vi "Move to New Position.vi"(7 "Curr Filter":i32, 8 "error in (no error)":errorcluster, 9 "Target Filter":i32, 10 "Filter Wheel (0:n-1)":i32, 11 "FW Arduino Control in":refnum<class "FW Arduino Control.lvclass">) -> (0 "error out":errorcluster, 1 "Actual Distance":i32[](array[numeric]), 2 "Log":string, 3 "FW Arduino Control out":refnum<class "FW Arduino Control.lvclass">)   [LabVIEW 2024, in "FW Arduino Control.lvclass"]
uses:
  FW Arduino Control.lvclass
  C:/Development/Prime-RIMAS/Filter Wheel/Filter Wheel Object/Filter Wheel.lvclass
  FW Arduino Control.lvclass/FW Arduino Control.ctl
panel:
  out "notches":i32
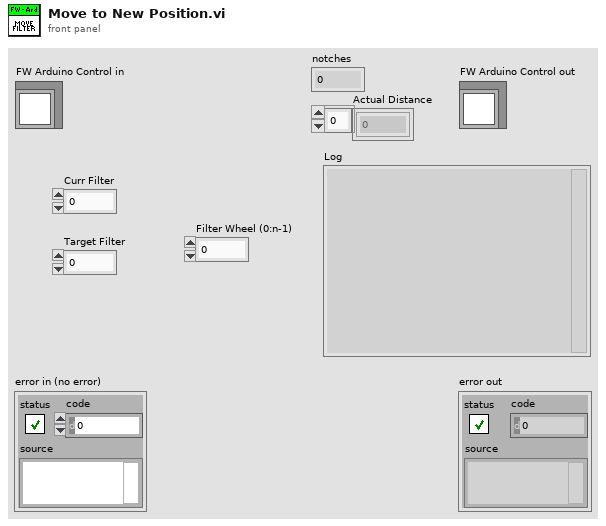
[diagram p1: front panel]
types:
  T1 = typedef "Filter Wheel Arduino Homing cluster.ctl" = cluster{"Direction (F: CW)":bool, "Speed":i32, "Accel":i32, "Min Distance":i32, "Short Leg":i32, "Error Cnts":i32}
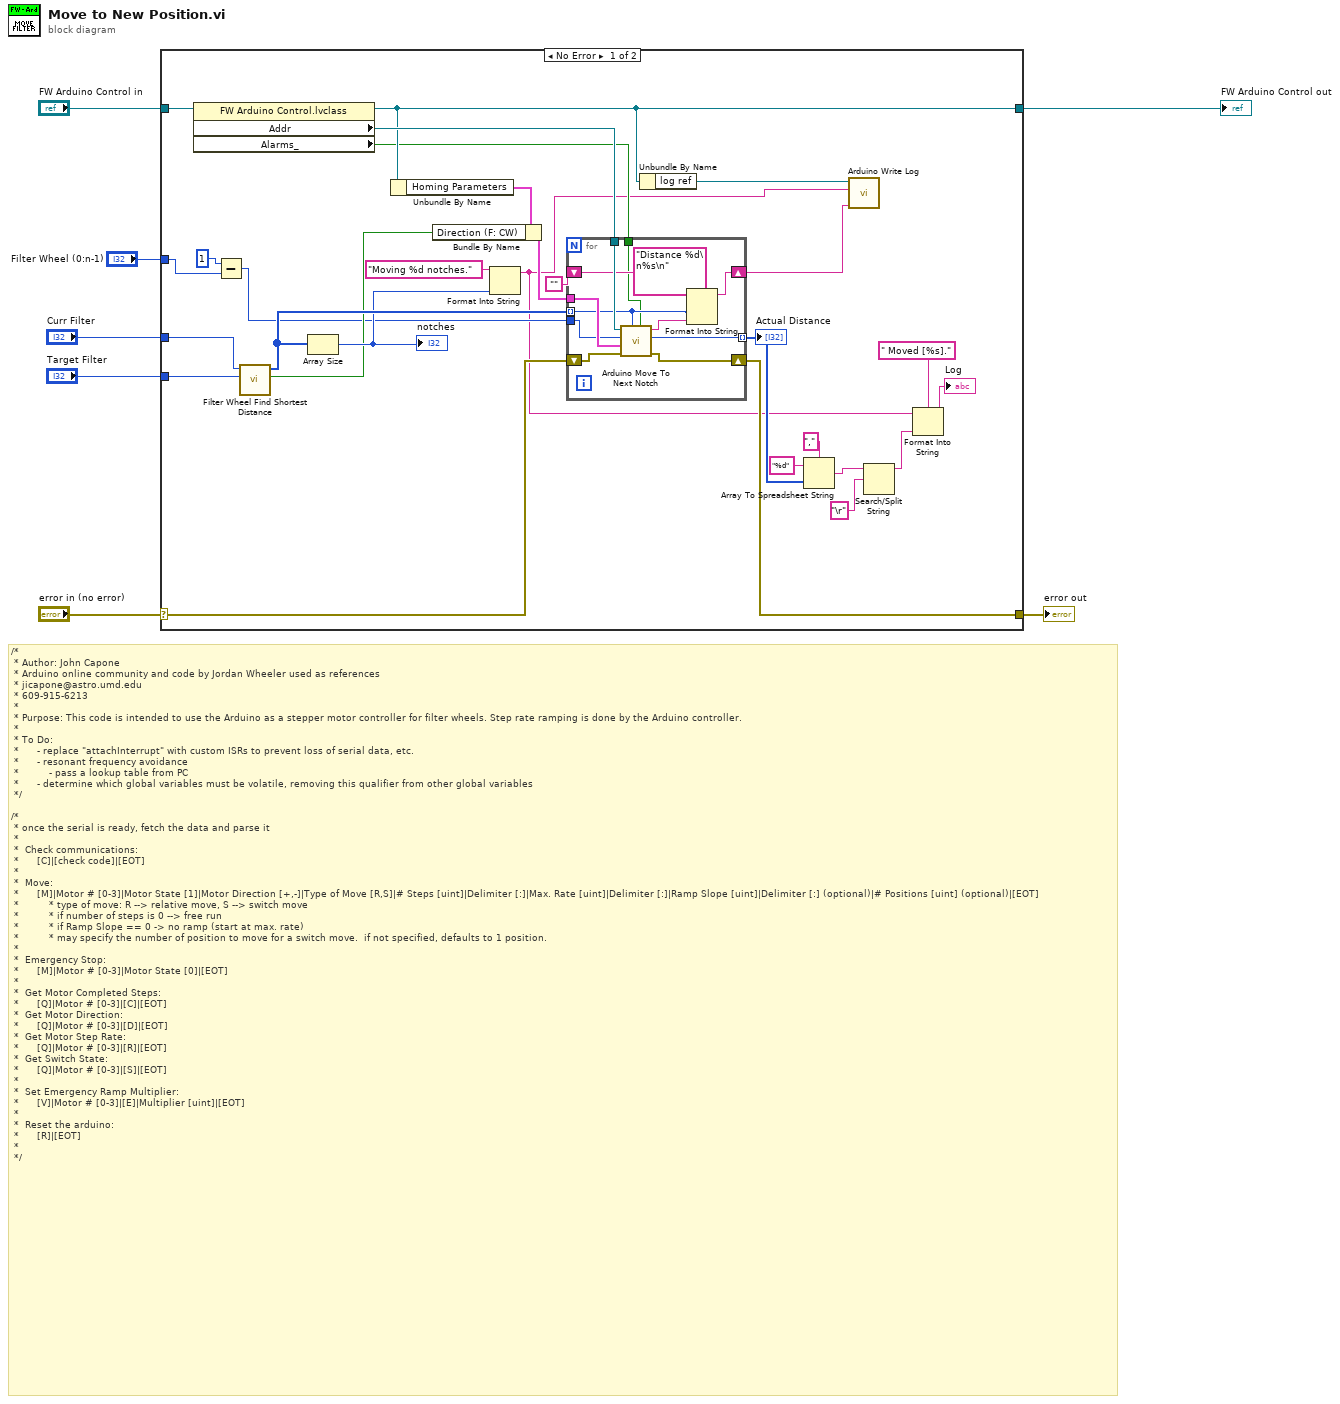
[diagram p0: block diagram]
diagram:
  # "/*\n * Author: John Capone\n * Arduino online community and code by Jordan Wheeler used as references\n * jicapone@astro.umd.edu\n * 609-915-6213\n * \n * Purpose: This code is intended to use the Arduino as a stepper motor controller for filter wheels. Step rate ramping is done by the Arduino controller.\n * \n * To Do:\n *      - replace \"attachInterrupt\" with custom ISRs to prevent loss of serial data, etc.\n *      - resonant frequency avoidance\n *          - pass a lookup table from PC\n *      - determine which global variables must be volatile, removing this qualifier from other global variables\n */\n\n/* \n * once the serial is ready, fetch the data and parse it\n *\n *  Check communications:\n *      [C]|[check code]|[EOT]\n *\n *  Move:\n *      [M]|Motor # [0-3]|Motor State [1]|Motor Direction [+,-]|Type of Move [R,S]|# Steps [uint]|Delimiter [:]|Max. Rate [uint]|Delimiter [:]|Ramp Slope [uint]|Delimiter [:] (optional)|# Positions [uint] (optional)|[EOT]\n *          * type of move: R --> relative move, S --> switch move\n *          * if number of steps is 0 --> free run\n *          * if Ramp Slope == 0 -> no ramp (start at max. rate)\n *          * may specify the number of position to move for a switch move.  if not specified, defaults to 1 position.\n *\n *  Emergency Stop:\n *      [M]|Motor # [0-3]|Motor State [0]|[EOT]\n *\n *  Get Motor Completed Steps:\n *      [Q]|Motor # [0-3]|[C]|[EOT]\n *  Get Motor Direction:\n *      [Q]|Motor # [0-3]|[D]|[EOT]\n *  Get Motor Step Rate:\n *      [Q]|Motor # [0-3]|[R]|[EOT]\n *  Get Switch State:\n *      [Q]|Motor # [0-3]|[S]|[EOT]\n *\n *  Set Emergency Ramp Multiplier:\n *      [V]|Motor # [0-3]|[E]|Multiplier [uint]|[EOT]\n *\n *  Reset the arduino:\n *      [R]|[EOT]\n *\n */"
  n1 = case shown="No Error" "error in (no error)" {
    selector: "error in (no error)" -> [w34 w50]
    tunnel: [w32 w50] -> w6
    tunnel: [w30 w49] -> w1
    tunnel: "FW Arduino Control in" -> [w36 w49]
    tunnel: "Filter Wheel (0:n-1)" -> [w20 _]
    tunnel: "Curr Filter" -> [w25 _]
    tunnel: "Target Filter" -> [w24 _]
    frame No Error {
      n2 = property class="FW Arduino Control.lvclass"(reference=w36) -> (reference out=w30:refnum<class "FW Arduino Control.lvclass">, "Addr"=w35:refnum<visa-resource-name>, "Alarms_"=w17:bool)  [unwired: 1 in, 1 out]
      n3 = Subtract(x=1, y=w20) -> (x-y=w18:i32)
      n4 = call "Filter Wheel Find Shortest Distance.vi"("Target Filter"=w24, "Curr Filter"=w25) -> ("forward?"=w21:bool, "Notches"=w23:i32[])  [unwired: 8 in]
      n5 = Array Size(array=w23) -> (size(s)=w22:i32)
      "notches" <- w22
      n6 = Unbundle By Name(w30) -> ("Homing Parameters"=w33:T1)
      n7 = Bundle By Name(cluster=w33, "Direction (F: CW)"=w21) -> (w26:T1)
      n8 = Format Into String(format string="Moving %d notches.", w22) -> (resulting string=w13:string)  [unwired: 2 in, 1 out]
      n9 = for {
        tunnel: w35 -> [w48]
        tunnel: w26 -> [w47]
        tunnel: w18 -> [w46]
        shift-right: [w44] -> w32
        shift-left: w34 -> [w45]
        shift-right: [w42] -> w28
        shift-left: "" -> [w41]
        tunnel: w23 -> [w39] mode=indexing
        tunnel: w17 -> [w38]
        tunnel: [w37] -> w16 mode=indexing
        n10 = call "Arduino Move To Next Notch.vi"("Ignore Alarm"=w38, "Distance"=w39, "error in"=w45, "Homing Parameters"=w47, "Motor"=w46, "Addr"=w48) -> ("error out"=w44:errorcluster, "Actual distance"=w37:i32, "Log"=w40:string)  [unwired: 3 in]
        n11 = Format Into String(format string="Distance %d\n%s\n", initial string=w41, w39, w40) -> (resulting string=w42:string)  [unwired: 1 in, 1 out]
      }
      "Actual Distance" <- w16
      n12 = Unbundle By Name(w30) -> ("log ref"=w29:refnum<file>)
      n13 = Array To Spreadsheet String(delimiter (Tab)=",", array=w16, 3:"%d" ("format string")) -> (spreadsheet string=w9:string)
      n14 = call "Arduino Write Log.vi"("Arduino data"=w28, "Message"=w13, "log ref"=w29) -> ()  [unwired: 9 in]
      n15 = Search/Split String(string=w9, search string/char (-)="\r") -> (substring before match=w8:string)  [unwired: 1 in, 2 out]
      n16 = Format Into String(format string=" Moved [%s].", initial string=w13, w8) -> (resulting string=→"Log":string)  [unwired: 1 in, 1 out]
    }
    frame Error {
    }
  }
  "error out" <- w6
  "FW Arduino Control out" <- w1
